vi "2283_driveTrainTest.vi"(4 "p":dbl(knob) scale=0.0..1.0, 5 "g":dbl(knob) scale=-1.0..1.0, 6 "x":dbl(knob) scale=-1.0..1.0, 7 "y":dbl(knob) scale=-1.0..1.0) -> (0 "d2":dbl(slide) scale=-1.0..1.0, 1 "i2":dbl(slide) scale=-1.0..1.0, 2 "d1":dbl(slide) scale=-1.0..1.0, 3 "i1":dbl(slide) scale=-1.0..1.0)   [LabVIEW 2014]
panel:
  out "result 2":dbl
  out "result":dbl
  in  "Boton 4":bool
  in  "Boton 3":bool
  in  "Boton 2":bool
  in  "Boton 1":bool
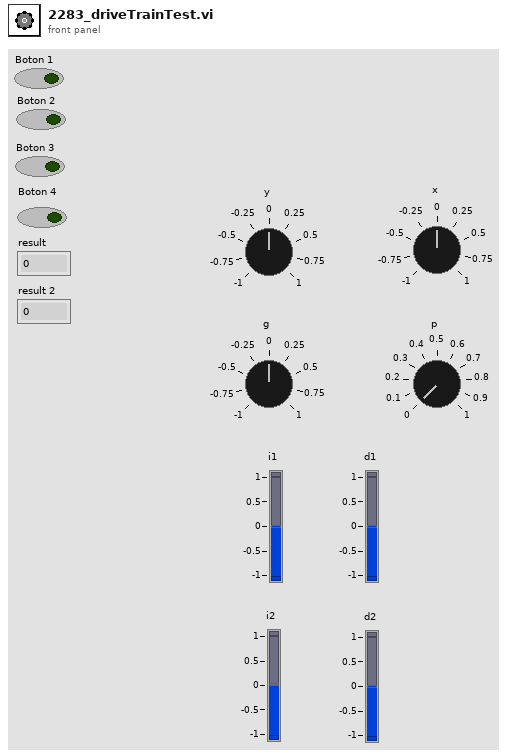
[diagram p1: front panel]
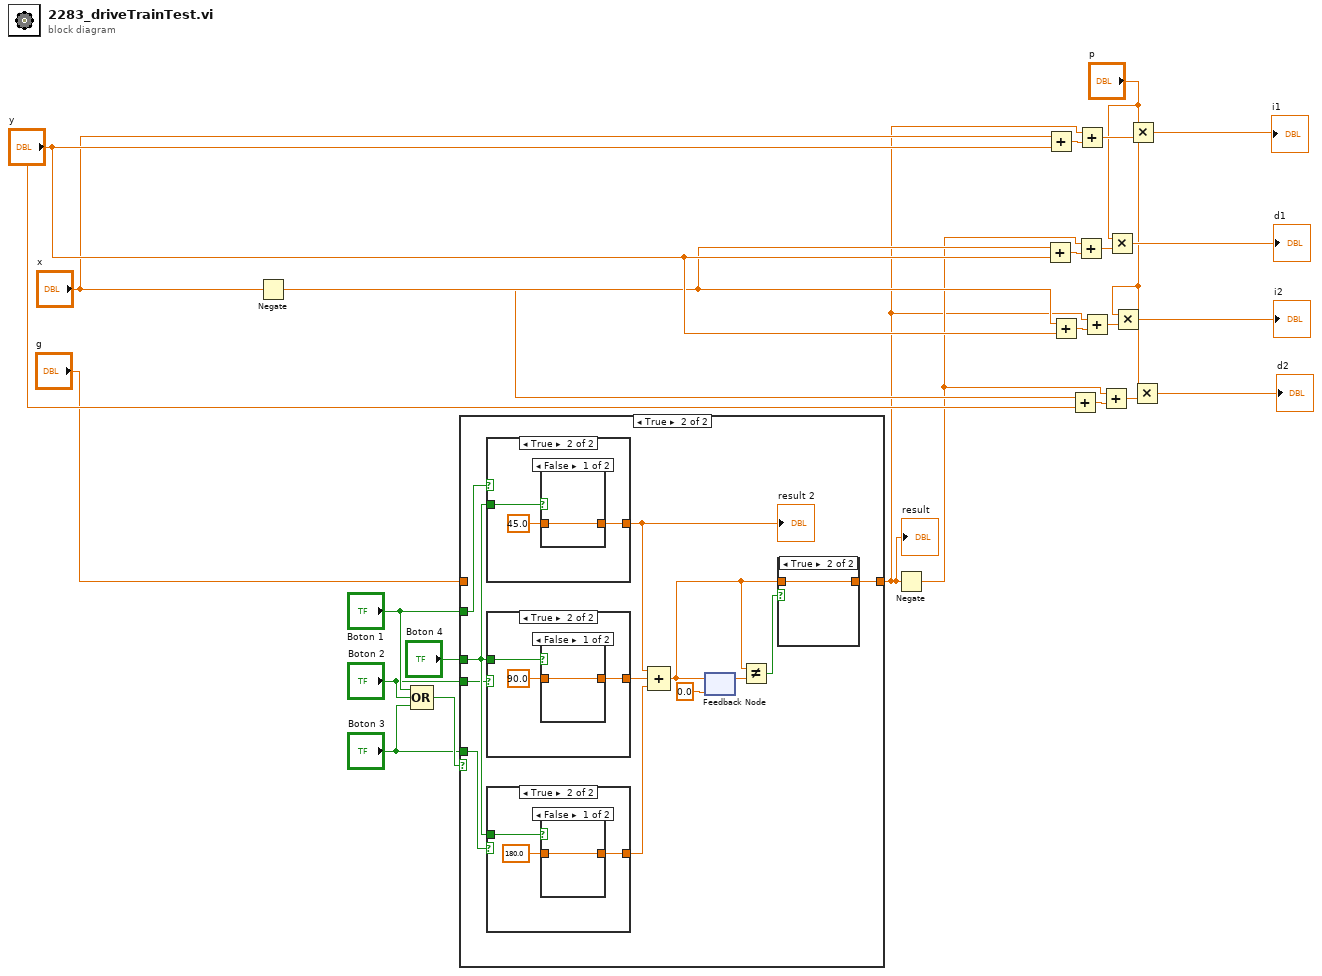
[diagram p0: block diagram]
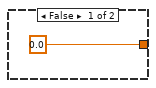
[diagram p3: hidden frame]
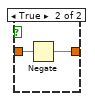
[diagram p4: hidden frame]
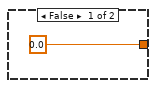
[diagram p5: hidden frame]
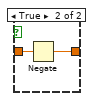
[diagram p6: hidden frame]
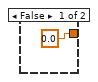
[diagram p7: hidden frame]
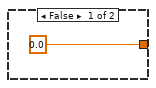
[diagram p8: hidden frame]
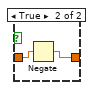
[diagram p9: hidden frame]
diagram:
  n1 = Negate(x="x") -> (-x=w19:dbl)
  n2 = Compound Arithmetic op=OR("Boton 1", "Boton 2", "Boton 3") -> (w6:bool)
  n3 = case shown="True" w6 {
    tunnel: "g" -> [w25 _]
    tunnel: [w25 w33] -> w5
    tunnel: "Boton 1" -> [_ w29]
    tunnel: "Boton 3" -> [_ w28]
    tunnel: "Boton 4" -> [_ w27]
    tunnel: "Boton 2" -> [_ w26]
    frame False {
    }
    frame True {
      n4 = case shown="True" w29 {
        tunnel: w27 -> [_ w55]
        tunnel: [0.0 ("g output") w56] -> w30
        frame False {
        }
        frame True {
          n5 = case shown="False" w55 {
            tunnel: [w58 w59] -> w56
            tunnel: 45.0 ("angulo deseado") -> [w58 w60]
            frame False {
            }
            frame True {
              n6 = Negate(x=w60) -> (-x=w59:dbl)
            }
          }
        }
      }
      "result 2" <- w30
      n7 = case shown="True" w26 {
        tunnel: w27 -> [_ w46]
        tunnel: [0.0 ("g output") w47] -> w32
        frame False {
        }
        frame True {
          n8 = case shown="False" w46 {
            tunnel: [w49 w50] -> w47
            tunnel: 90.0 ("angulo deseado") -> [w49 w51]
            frame False {
            }
            frame True {
              n9 = Negate(x=w51) -> (-x=w50:dbl)
            }
          }
        }
      }
      n10 = case shown="True" w28 {
        tunnel: w27 -> [_ w39]
        tunnel: [0.0 ("g output") w40] -> w31
        frame False {
        }
        frame True {
          n11 = case shown="False" w39 {
            tunnel: [w42 w43] -> w40
            tunnel: 180.0 ("angulo deseado") -> [w42 w44]
            frame False {
            }
            frame True {
              n12 = Negate(x=w44) -> (-x=w43:dbl)
            }
          }
        }
      }
      n13 = Compound Arithmetic op=ADD(w30, w32, w31) -> (w34:dbl)
      n14 = feedback-in #1(w34) -> ()
      n15 = feedback #1(0.0) -> (w36:dbl)
      n16 = Not Equal?(x=w34, y=w36) -> (x != y?=w35:bool)
      n17 = case shown="True" w35 {
        tunnel: w34 -> [_ w53]
        tunnel: [0.0 w53] -> w33
        frame False {
        }
        frame True {
        }
      }
    }
  }
  "result" <- w5
  n18 = Negate(x=w5) -> (-x=w17:dbl)
  n19 = Add(x=w19, y="y") -> (x+y=w23:dbl)
  n20 = Add(x="x", y="y") -> (x+y=w24:dbl)
  n21 = Add(x=w19, y="y") -> (x+y=w22:dbl)
  n22 = Add(x="x", y="y") -> (x+y=w20:dbl)
  n23 = Add(x=w17, y=w23) -> (x+y=w14:dbl)
  n24 = Add(x=w5, y=w24) -> (x+y=w13:dbl)
  n25 = Add(x=w5, y=w22) -> (x+y=w15:dbl)
  n26 = Add(x=w17, y=w20) -> (x+y=w16:dbl)
  n27 = Multiply(x="p", y=w14) -> (x*y=→"d1":dbl)
  n28 = Multiply(x="p", y=w15) -> (x*y=→"i2":dbl)
  n29 = Multiply(x="p", y=w13) -> (x*y=→"i1":dbl)
  n30 = Multiply(x="p", y=w16) -> (x*y=→"d2":dbl)
